vi "Database Command Create.vi"(7 "stored procedure? (F)":bool, 8 "error in (no error)":errorcluster caption="错误输入（无错误）", 9 "CommandTimeout":i32, 10 "SQL query":string, 11 "Database Command 输入":refnum<class "Database Command.lvclass"> caption="DNL_LabVIEW Object in") -> (0 "error out":errorcluster caption="错误输出", 3 "Database Command 输出":refnum<class "Database Command.lvclass"> caption="DNL_LabVIEW Object out")   [LabVIEW 2011, in "Database Command.lvclass"]
uses:
  Database Command.lvclass
  Database Command.lvclass/Database Command.ctl
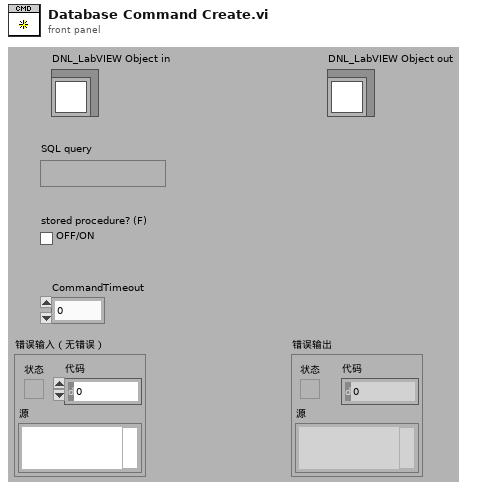
[diagram p1: front panel]
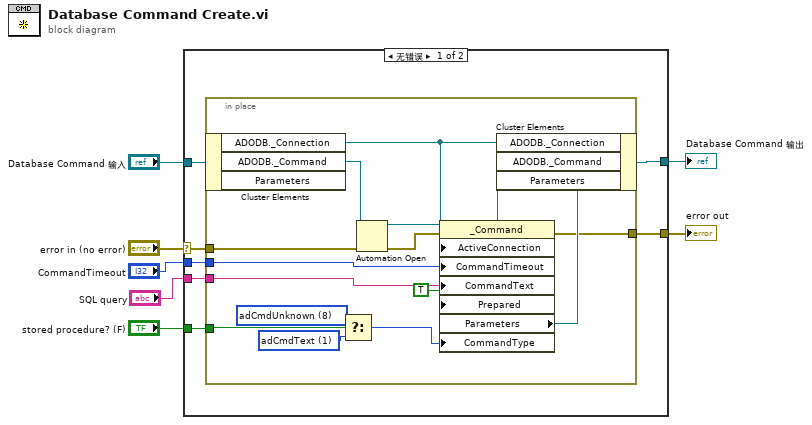
[diagram p0: block diagram]
diagram:
  n1 = case shown="无错误" "error in (no error)" {
    selector: "error in (no error)" -> [w12 w31]
    tunnel: [w9 w31] -> w6
    tunnel: [w13 w30] -> w4
    tunnel: "Database Command 输入" -> [w14 w30]
    tunnel: "stored procedure? (F)" -> [w11 _]
    tunnel: "SQL query" -> [w10 _]
    tunnel: "CommandTimeout" -> [w8 _]
    frame No Error {
      n2 = in-place {
        in-place-border: w12 -> [w29]
        in-place-border: w11 -> [w26]
        in-place-border: w10 -> [w23]
        in-place-border: [w19] -> w9
        in-place-border: w8 -> [w15]
        w28 = 1 items=["adCmdUnspecified"=-1, "adCmdUnknown"=8, "adCmdText"=1, "adCmdTable"=2, "adCmdStoredProc"=4, "adCmdFile"=256, "adCmdTableDirect"=512] ("CommandType")
        w27 = 8 items=["adCmdUnspecified"=-1, "adCmdUnknown"=8, "adCmdText"=1, "adCmdTable"=2, "adCmdStoredProc"=4, "adCmdFile"=256, "adCmdTableDirect"=512] ("CommandType")
        n3 = in-place-cluster #1(w14) -> ("ADODB._Connection"=w20:refnum<k7>, "ADODB._Command"=w24:refnum<k7>)  [unwired: 1 out]
        n4 = Select(t=w27, s=w26, f=w28) -> (s? t:f=w17:i32)
        n5 = Automation Open(error in (no error)=w29, Automation Refnum=w24) -> (Automation Refnum=w16:refnum<k7>, error out=w25:errorcluster)  [unwired: 2 in]
        n6 = property class="_Command"(reference=w16, error in=w25, "ActiveConnection"=w20, "CommandTimeout"=w15, "CommandText"=w23, "Prepared"=TRUE, "CommandType"=w17) -> (reference out=w18:refnum<k7>, error out=w19:errorcluster, "Parameters"=w21:refnum<k7>)
        n7 = in-place-cluster #1("ADODB._Connection"=w20, "ADODB._Command"=w18, "Parameters"=w21) -> (w13:refnum<class "Database Command.lvclass">)
      }
    }
    frame Error {
    }
  }
  "error out" <- w6
  "Database Command 输出" <- w4
